vi "Data Compile (Tree).vi"(8 "error in (no error)":errorcluster, 9 "Tree in":refnum<data-value>, 10 "Expression":string, 11 "Data DVR in":refnum<data-value>) -> (0 "error out":errorcluster, 1 "Tree out":refnum<data-value>, 2 "Data out":refnum<data-value>, 3 "Data DVR out":refnum<data-value>)   [LabVIEW 2010, in "MDSplus.lvlib"]
doc: "Static method which compiles the expression (via TdiCompile()) and returns the object instance correspondind to the compiled expression."
uses:
  <vilib>/MDSplus/Library/MDSplus.lvlib
  <vilib>/MDSplus/Classes/Tree_Class/Tree.lvclass
  <vilib>/MDSplus/Classes/Data_Class/Data.lvclass
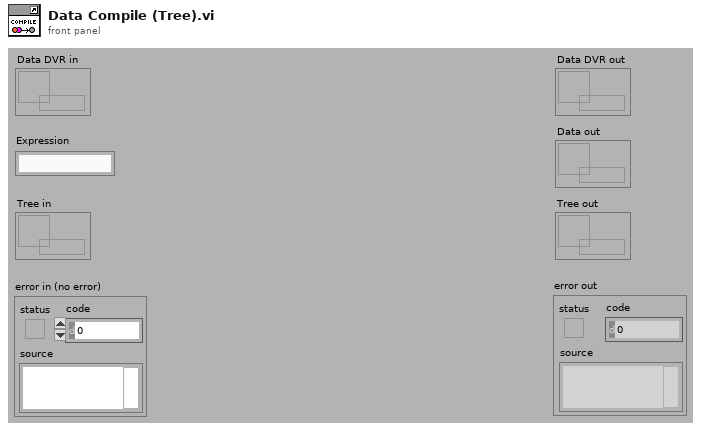
[diagram p1: front panel]
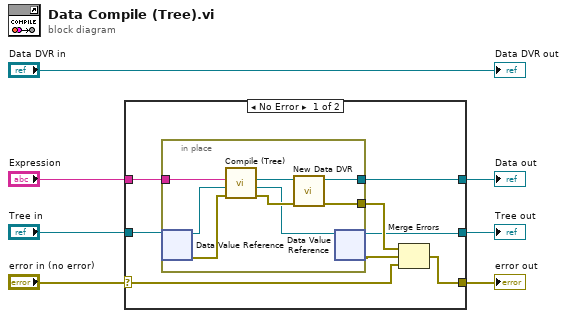
[diagram p0: block diagram]
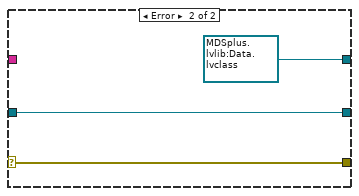
[diagram p2: hidden frame]
diagram:
  n1 = case shown="No Error" "error in (no error)" {
    selector: "error in (no error)" -> [w15 w26]
    tunnel: [w14 w26] -> w4
    tunnel: [w12 refnum<data-value> refnum ("TreeNode DVR out")] -> w2
    tunnel: "Expression" -> [w13 _]
    tunnel: "Tree in" -> [w10 w24]
    tunnel: [w9 w24] -> w3
    frame No Error {
      n2 = in-place {
        in-place-border: [w22] -> w11
        in-place-border: w13 -> [w20]
        in-place-border: [w23] -> w12
        n3 = in-place-dvr #1(w10) -> (w18:refnum<class "Tree.lvclass">, w17:errorcluster)
        n4 = call <vilib>:"Compile (Tree).vi"("error in (no error)"=w17, "Tree in"=w18, "Expression"=w20) -> ("error out"=w21:errorcluster, "Tree out"=w16:refnum<class "Tree.lvclass">, "Returned data out"=w19:refnum<class "Data.lvclass">)  [unwired: 5 in, 1 out]
        n5 = call <vilib>:"New Data DVR.vi"("error in (no error)"=w21, "Data in"=w19) -> ("error out"=w22:errorcluster, "Data DVR out"=w23:refnum<data-value>)  [unwired: 8 in]
        n6 = in-place-dvr #1(w16) -> (w9:refnum<data-value>, w8:errorcluster)
      }
      n7 = Merge Errors(w11, w8, w15) -> (w14:errorcluster)
    }
    frame Error {
    }
  }
  "error out" <- w4
  "Tree out" <- w3
  "Data out" <- w2
  "Data DVR out" <- "Data DVR in"
